vi "Template.vi"(8 "Error IN":errorcluster, 11 "HEKAdat.lvclass IN":refnum<class "HEKAdat.lvclass">) -> (0 "Error OUT":errorcluster, 3 "HEKAdat.lvclass OUT":refnum<class "HEKAdat.lvclass">)   [LabVIEW 2017, in "HEKAdat.lvclass"]
uses:
  HEKAdat.lvclass
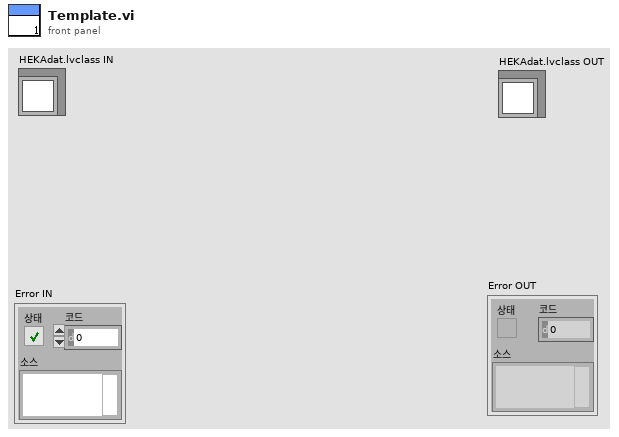
[diagram p1: front panel]
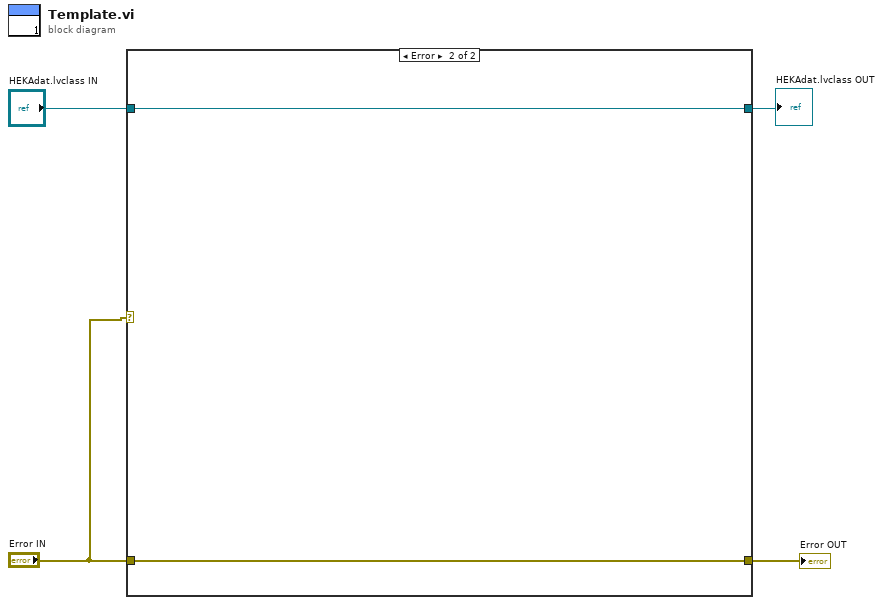
[diagram p0: block diagram]
diagram:
  n1 = case shown="Error" "Error IN" {
    tunnel: "Error IN" -> [w6 w7]
    tunnel: [w6 w7] -> w3
    tunnel: "HEKAdat.lvclass IN" -> [w5 w8]
    tunnel: [w5 w8] -> w1
    frame No Error {
    }
    frame Error {
    }
  }
  "HEKAdat.lvclass OUT" <- w1
  "Error OUT" <- w3
